vi "Logging Message Loop.vi"(8 "error in (no error)":errorcluster, 10 "data queue in":refnum<queue>, 11 "Message Queues":T1) -> (0 "error out":errorcluster)   [LabVIEW 2026, in "Logging.lvlib"]
doc: "The message loop subVI to handle messages pertaining to logging data."
uses:
  Logging.lvlib
  support/Message Queue/All Message Queues.ctl
  support/Message Queue/Message Cluster.ctl
  controls/NotifierAndDataQueue.ctl
  controls/WaveformChartData.ctl
  Logging Configuration.ctl
  Logging State.ctl
  support/Message Queue/Enqueue Message (Single).vi
  <vilib>/Utility/error.llb/Error Cluster From Error Code.vi
  <vilib>/ErrorRing/Error Ring.xnode
  support/Message Queue/Message Queue.lvlib
  Settings/Settings.lvlib
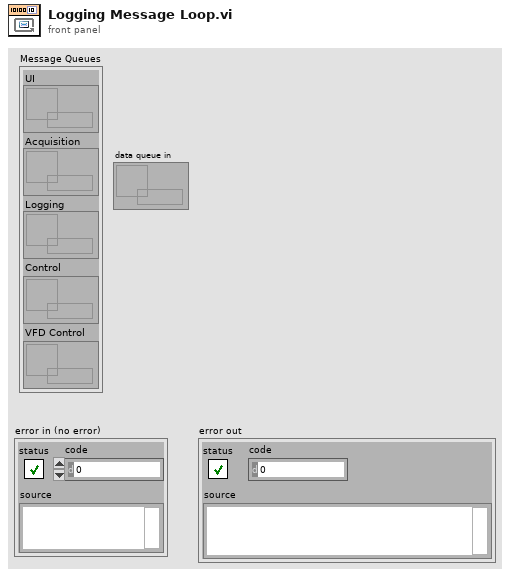
[diagram p1: front panel]
types:
  T1 = typedef "Message Queue.lvlib/All Message Queues.ctl" = cluster{"UI":refnum<queue>, "Acquisition":refnum<queue>, "Logging":refnum<queue>, "Control":refnum<queue>, "VFD Control":refnum<queue>}
  T2 = typedef "Logging.lvlib/Logging State.ctl" = cluster{"State":enum16{"Logging", "Not Logging", "Idle"}, "Samples to Save":u32, "Force Trigger":bool}
  T3 = typedef "Logging.lvlib/Logging Configuration.ctl" = cluster{"Log File Base Path":path, "TDMS File Reference":refnum<k34>, "File Name":string, "Headers To Write":string[]}
  T4 = enum16{"open", "open or create", "create or replace", "create", "open (read-only)"}
  T5 = typedef "NotifierAndDataQueue.ctl" = cluster{"Ai0":dbl, "Ai1":dbl, "Ai2":dbl, "Ai3":dbl, "Ai4":dbl, "Ai5":dbl, "Ai6":dbl, "Ai7":dbl, "Belt Slip?":bool, "P0.1":bool, "P0.2":bool, "P0.3":bool, "P0.4":bool, "P0.5":bool, "P0.6":bool, "P0.7":bool, "2D Numeric Data":dbl[][], "String 2":string, "String 1":string, "Waveform Chart Data":T6, "Live Pulley Ratio":dbl, "Data Table":string[][]}
  T6 = typedef "Settings.lvlib/WaveformChartData.ctl" = cluster{"DUT Vacuum":dbl, "Motor RPM":dbl, "DUT RPM":dbl, "Tank Vacuum":dbl}
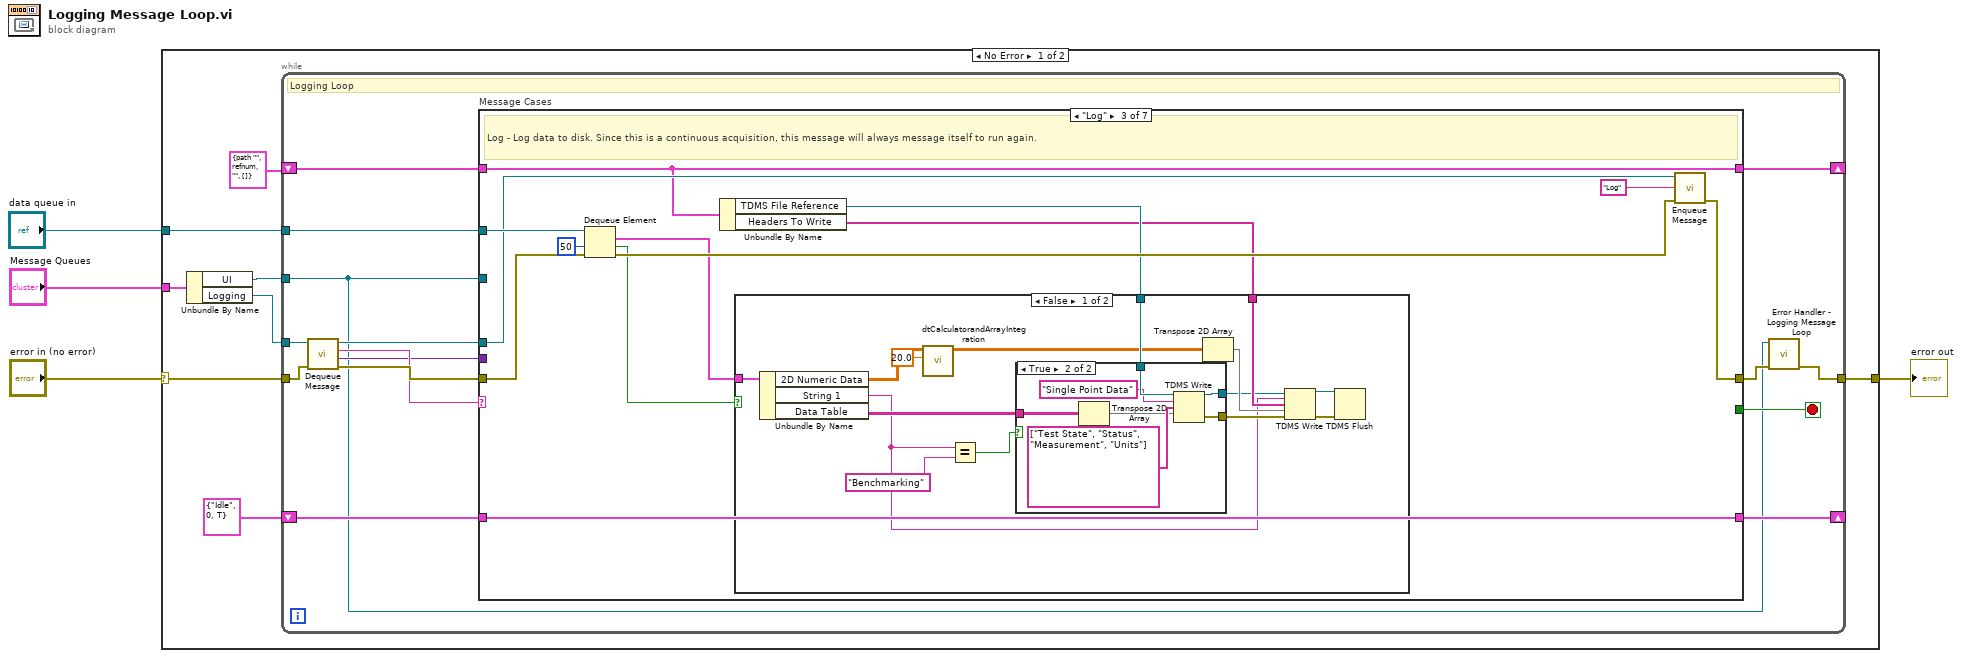
[diagram p0: block diagram]
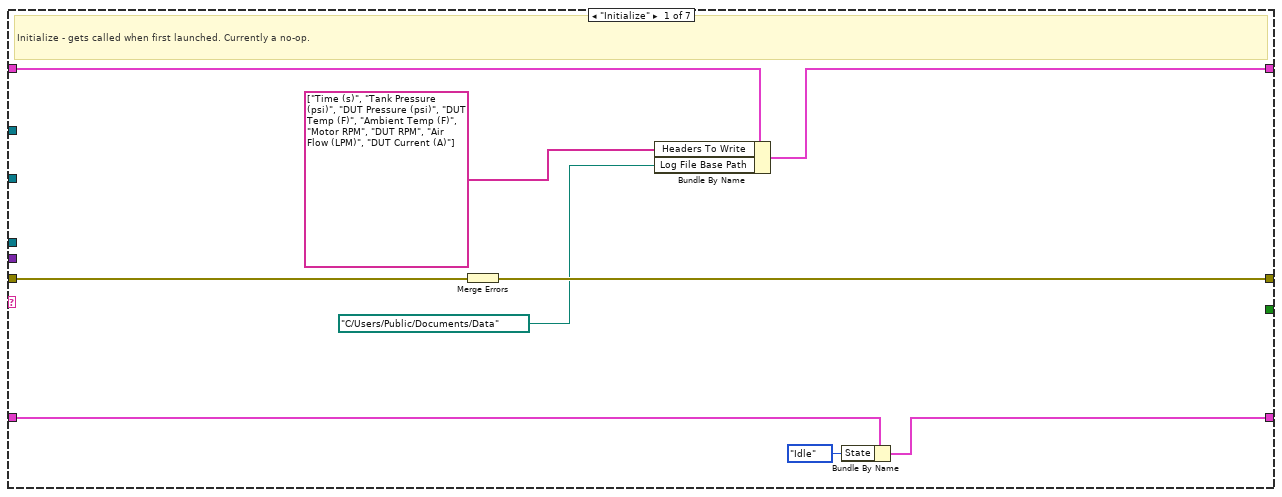
[diagram p2: hidden frame]
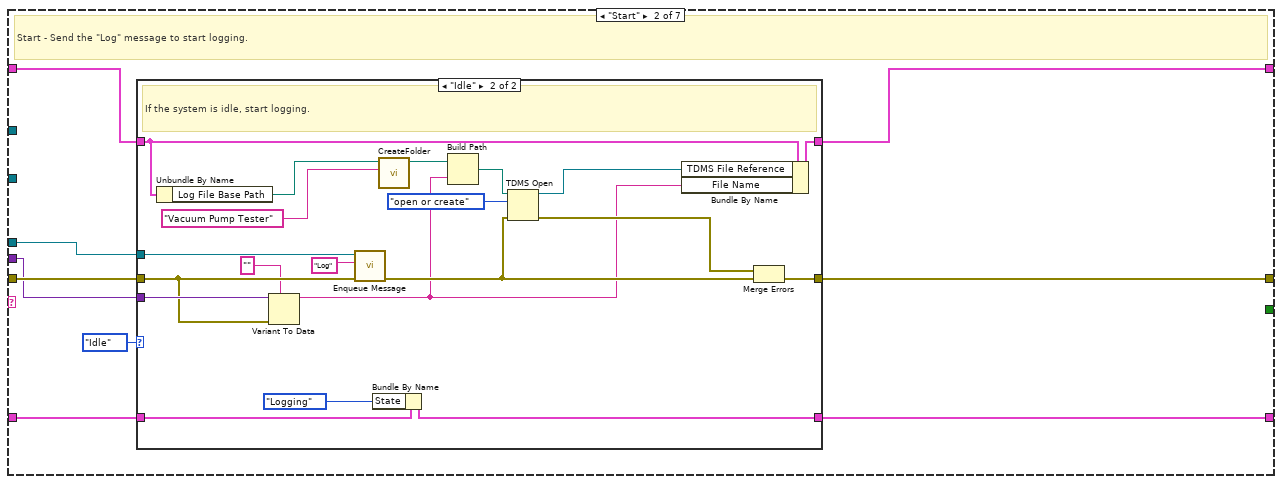
[diagram p3: hidden frame]
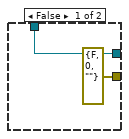
[diagram p5: hidden frame]
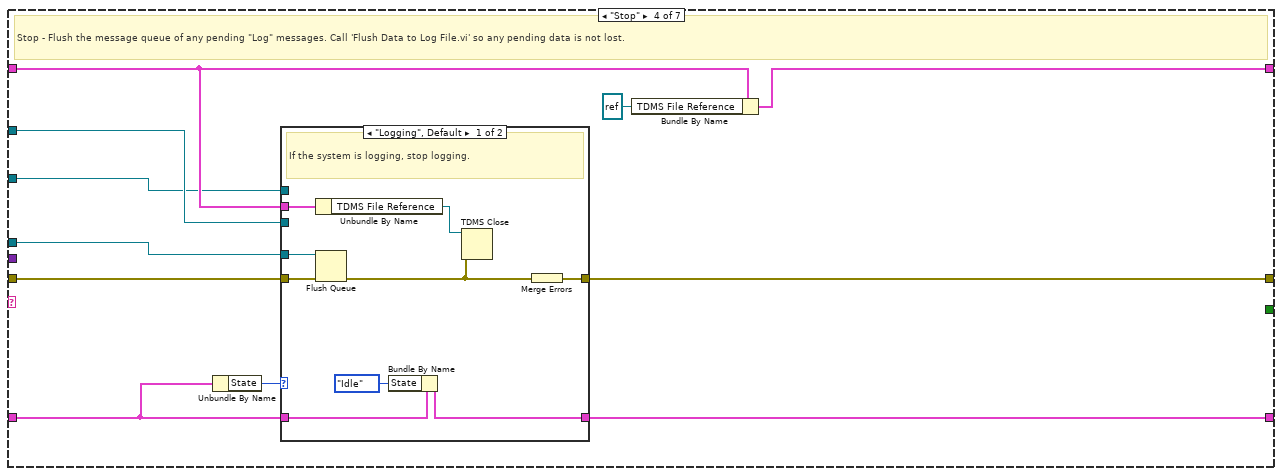
[diagram p7: hidden frame]
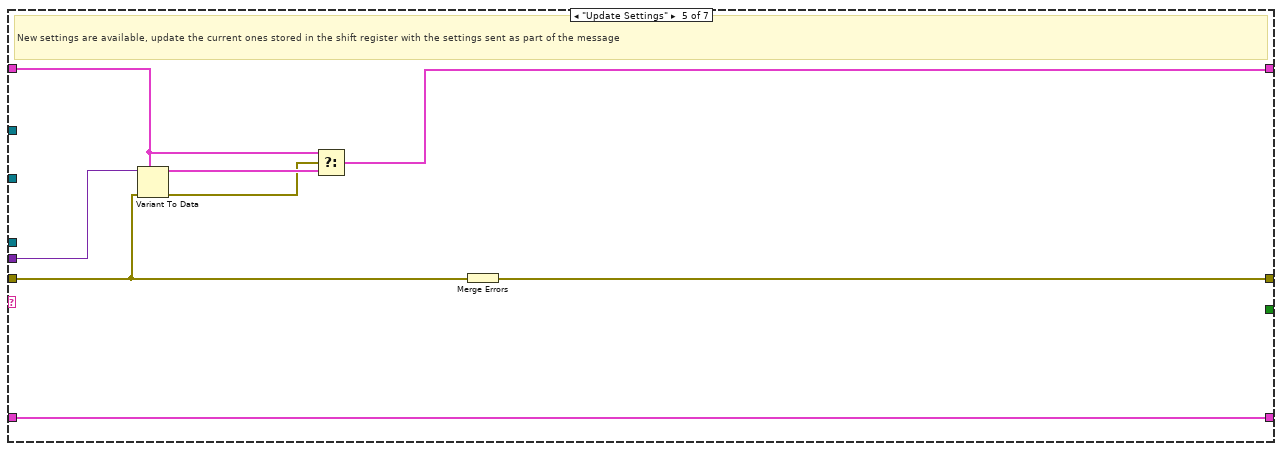
[diagram p9: hidden frame]
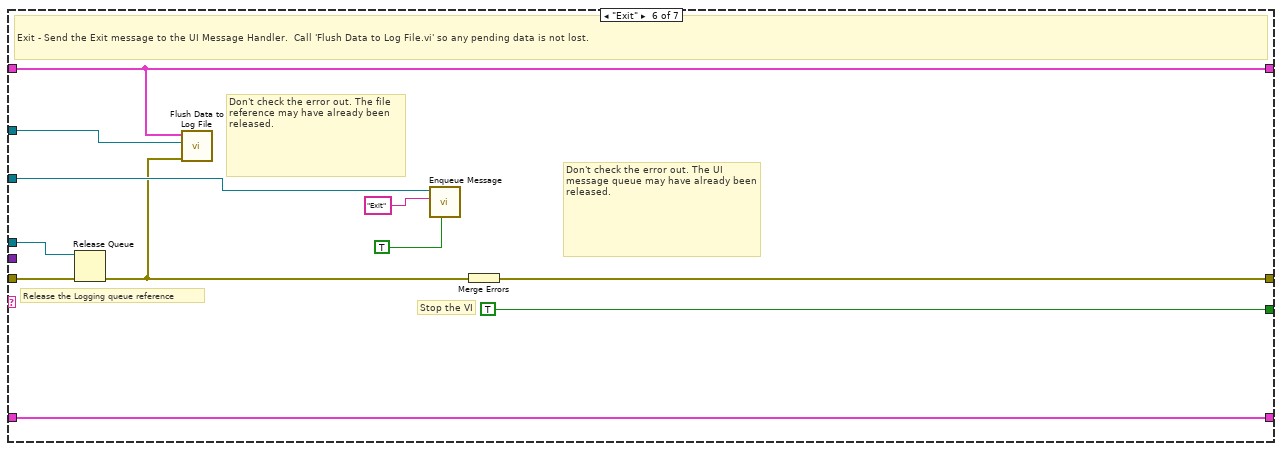
[diagram p10: hidden frame]
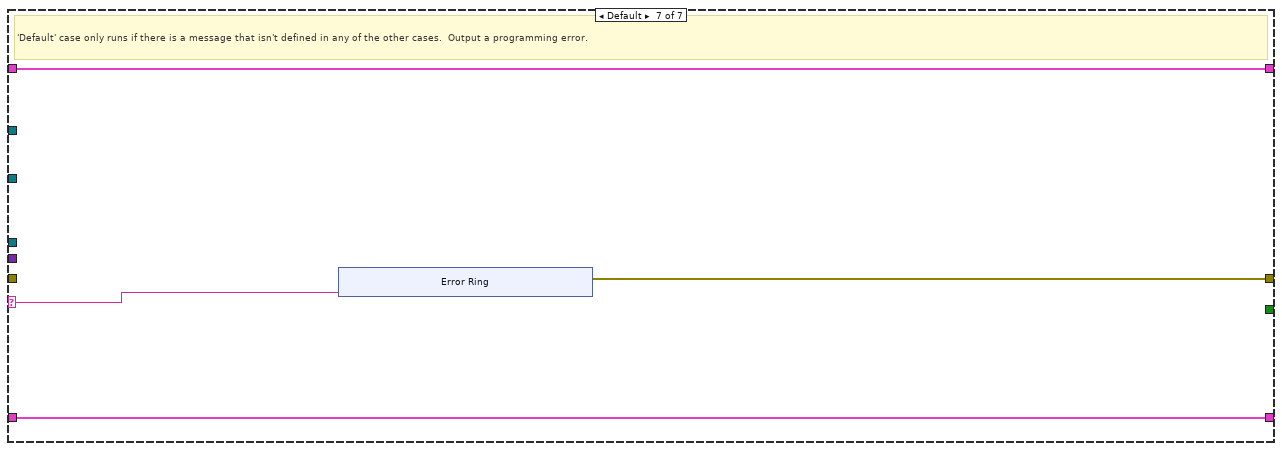
[diagram p11: hidden frame]
diagram:
  n1 = case shown="No Error" "error in (no error)" {
    selector: "error in (no error)" -> [w8 w158]
    tunnel: "Message Queues" -> [w12 _]
    tunnel: [w10 w158] -> w3
    tunnel: "data queue in" -> [w7 _]
    frame No Error {
      n2 = Unbundle By Name(w12) -> ("UI"=w6:refnum<queue>, "Logging"=w11:refnum<queue>)
      n3 = while {
        tunnel: w11 -> [w19]
        shift-right: [w26] -> _
        shift-left: T3 {"Log File Base Path"=path "", "TDMS File Reference"=refnum, "File Name"="", "Headers To Write"=[]} ("Logging Configuration") -> [w27]
        tunnel: w6 -> [w14]
        tunnel: w7 -> [w13]
        shift-right: [w17] -> _
        shift-left: T2 {"State"=enum."Idle", "Samples to Save"=0, "Force Trigger"=TRUE} -> [w18]
        tunnel: w8 -> [w24]
        tunnel: [w15] -> w10
        stop <- w25 stop-if-true
        # "Logging Loop"
        n4 = call "Dequeue Message.vi"("error in (no error)"=w24, "Message Queue"=w19) -> ("error out"=w23:errorcluster, "Message Data"=w21:variant, "Message"=w22:string, "dup Message Queue"=w20:refnum<queue>)  [unwired: 6 in]
        n5 = case "Message Cases" shown="\"Log\"" w22 {
          selector: w22 -> [_ _ _ _ _ _ w147]
          tunnel: w20 -> [_ w44 w77 w114 _ w140 _]
          tunnel: w23 -> [w35 w43 w79 w115 w129 w143 _]
          tunnel: [w36 w45 w81 w116 w135 w145 w148] -> w16
          tunnel: w27 -> [w31 w42 w74 w111 w133 w139 w150]
          tunnel: [w30 w41 w74 w113 w130 w139 w150] -> w26
          tunnel: [_ _ _ _ _ TRUE _] -> w25
          tunnel: w21 -> [_ w38 _ _ w134 _ _]
          tunnel: w14 -> [_ _ _ w109 _ w144 _]
          tunnel: w13 -> [_ _ w78 w110 _ w136 _]
          tunnel: w18 -> [w34 w39 w76 w107 w128 w137 w149]
          tunnel: [w33 w40 w76 w106 w128 w137 w149] -> w17
          frame "Initialize" {
            # "Initialize - gets called when first launched. Currently a no-op."
            n6 = Merge Errors(w35) -> (w36:errorcluster)
            n7 = Bundle By Name(cluster=w31, "Headers To Write"=string[] ["Time (s)", "Tank Pressure (psi)", "DUT Pressure (psi)", "DUT Temp (F)", "Ambient Temp (F)", "Motor RPM", "DUT RPM", "Air Flow (LPM)", "DUT Current (A)"], "Log File Base Path"=path "C:/Users/Public/Documents/Data") -> (w30:T3)
            n8 = Bundle By Name(cluster=w34, "State"=enum16{"Logging", "Not Logging", "Idle"}."Idle") -> (w33:T2)
          }
          frame "Start" {
            # "Start - Send the \"Log\" message to start logging."
            n9 = case shown="\"Idle\"" enum16{"Logging", "Not Logging", "Idle"}."Idle" ("State") {
              tunnel: [w47 w68] -> w45
              tunnel: w44 -> [_ w67]
              tunnel: w43 -> [w47 w52]
              tunnel: w42 -> [w48 w65]
              tunnel: [w48 w62] -> w41
              tunnel: w39 -> [w46 w58]
              tunnel: [w46 w57] -> w40
              tunnel: w38 -> [_ w53]
              frame "Logging", Default {
                # "The system is already running. Ignore the \"Start\" message."
              }
              frame "Idle" {
                # "If the system is idle, start logging."
                n10 = Unbundle By Name(w65) -> ("Log File Base Path"=w55:path)
                n11 = Variant To Data(error in=w52, type="", Variant=w53) -> (data=w50:string)  [unwired: 1 out]
                n12 = call-poly "Enqueue Message.vi"("error in (no error)"=w52, "Message"="Log", "Message Queue"=w67) -> ("error out"=w60:errorcluster)  [unwired: 7 in, 1 out]
                n13 = Bundle By Name(cluster=w58, "State"=enum16{"Logging", "Not Logging"}."Logging") -> (w57:T2)
                n14 = call "CreateFolder.vi"("Folder Name"="Vacuum Pump Tester", "path (use dialog)"=w55) -> ("created path"=w54:path)  [unwired: 9 in]
                n15 = Build Path(base path=w54, name or relative path=w50) -> (appended path=w63:path)
                n16 = TDMS Open(8:w60, 10:T4."open or create" ("operation (0:open)"), 11:w63) -> (0:w59:errorcluster, 3:w64:refnum<k34>)  [unwired: 4 in]
                n17 = Bundle By Name(cluster=w65, "TDMS File Reference"=w64, "File Name"=w50) -> (w62:T3)
                n18 = Merge Errors(w59, w60) -> (w68:errorcluster)
              }
            }
          }
          frame "Log" {
            # "Log - Log data to disk. Since this is a continuous acquisition, this message will always message itself to run again."
            n19 = Dequeue Element(queue=w78, timeout in ms (-1)=50, error in (no error)=w79) -> (element=w73:T5, timed out?=w70:bool, error out=w75:errorcluster)  [unwired: 1 out]
            n20 = Unbundle By Name(w74) -> ("TDMS File Reference"=w72:refnum<k34>, "Headers To Write"=w69:string[])
            n21 = case shown="False" w70 {
              tunnel: w73 -> [w95 _]
              tunnel: w72 -> [w91 _]
              tunnel: w69 -> [w96 _]
              frame False {
                n22 = Unbundle By Name(w95) -> ("2D Numeric Data"=w87:dbl[][], "String 1"=w83:string, "Data Table"=w88:string[][])
                n23 = call "dtCalculatorandArrayIntegration.vi"("Sampling Rate"=20.0, "Data Input"=w87) -> ("output array"=w86:dbl[][])  [unwired: 9 in]
                n24 = Equal?(x=w83, y="Benchmarking") -> (x = y?=w84:bool)
                n25 = case shown="True" w84 {
                  tunnel: w91 -> [w98 w105]
                  tunnel: [w98 w104] -> w90
                  tunnel: [errorcluster {"status"=FALSE, "code"=0, "source"=""} ("error out") w103] -> w89
                  tunnel: w88 -> [_ w101]
                  frame False {
                  }
                  frame True {
                    n26 = Transpose 2D Array(2D array=w101) -> (transposed array=w99:string[][])
                    n27 = TDMS Write(0:w105, 5:"Single Point Data" ("group name in (Untitled)"), 7:string[] ["Test State", "Status", "Measurement", "Units"] ("Headers To Write"), 9:w99) -> (4:w104:refnum<k34>, 15:w103:errorcluster)  [unwired: 2 in, 2 out]
                  }
                }
                n28 = Transpose 2D Array(2D array=w86) -> (transposed array=w92:dbl[][])
                n29 = TDMS Write(0:w90, 5:w83, 7:w96, 9:w92, 11:w89) -> (4:w93:refnum<k34>, 15:w94:errorcluster)  [unwired: 1 in, 2 out]
                n30 = TDMS Flush(4:w94, 7:w93) -> ()  [unwired: 2 out]
              }
              frame True {
              }
            }
            n31 = call-poly "Enqueue Message.vi"("error in (no error)"=w75, "Message"="Log", "Message Queue"=w77) -> ("error out"=w81:errorcluster)  [unwired: 7 in, 1 out]
          }
          frame "Stop" {
            # "Stop - Flush the message queue of any pending \"Log\" messages. Call 'Flush Data to Log File.vi' so any pending data is not lost."
            n32 = Unbundle By Name(w107) -> ("State"=w108:enum16{"Logging", "Not Logging", "Idle"})
            n33 = case shown="\"Logging\", Default" w108 {
              tunnel: [w125 w127] -> w116
              tunnel: w115 -> [w124 w127]
              tunnel: w114 -> [w123 _]
              tunnel: w111 -> [w118 _]
              tunnel: w110 -> [_ _]
              tunnel: w109 -> [_ _]
              tunnel: w107 -> [w122 w126]
              tunnel: [w121 w126] -> w106
              frame "Logging", Default {
                # "If the system is logging, stop logging."
                n34 = Unbundle By Name(w118) -> ("TDMS File Reference"=w117:refnum<k34>)
                n35 = Flush Queue(queue=w123, error in (no error)=w124) -> (error out=w119:errorcluster)  [unwired: 2 out]
                n36 = Bundle By Name(cluster=w122, "State"=enum16{"Logging", "Not Logging", "Idle"}."Idle") -> (w121:T2)
                n37 = TDMS Close(8:w119, 11:w117) -> ()  [unwired: 2 out]
                n38 = Merge Errors(w119) -> (w125:errorcluster)
              }
              frame "Idle" {
                # "The system is already idle. Ignore the \"Stop\" message."
              }
            }
            n39 = Bundle By Name(cluster=w111, "TDMS File Reference"=refnum<k34> refnum ("tdms file out")) -> (w113:T3)
          }
          frame "Update Settings" {
            # "New settings are available, update the current ones stored in the shift register with the settings sent as part of the message"
            n40 = Variant To Data(error in=w129, type=w133, Variant=w134) -> (data=w132:T3, error out=w131:errorcluster)
            n41 = Select(t=w133, s=w131, f=w132) -> (s? t:f=w130:T3)
            n42 = Merge Errors(w129) -> (w135:errorcluster)
          }
          frame "Exit" {
            # "Don't check the error out. The file reference may have already been released."
            # "Release the Logging queue reference"
            # "Don't check the error out. The UI message queue may have already been released."
            # "Stop the VI"
            # "Exit - Send the Exit message to the UI Message Handler.  Call 'Flush Data to Log File.vi' so any pending data is not lost."
            n43 = Release Queue(queue=w140, error in (no error)=w143) -> (error out=w138:errorcluster)  [unwired: 1 in, 2 out]
            n44 = call "Flush Data to Log File.vi"("error in (no error)"=w138, "data queue in"=w136, "Logging Configuration"=w139) -> ()  [unwired: 8 in, 1 out]
            n45 = call-poly "Enqueue Message.vi"("Priority Message? (F)"=TRUE, "Message"="Exit", "Message Queue"=w144) -> ()  [unwired: 7 in, 2 out]
            n46 = Merge Errors(w138) -> (w145:errorcluster)
          }
          frame Default {
            # "'Default' case only runs if there is a message that isn't defined in any of the other cases.  Output a programming error."
            n47 = xnode "Error Ring"("parameter 0"=w147) -> ("error out"=w148:errorcluster)
          }
        }
        n48 = call "Error Handler - Logging Message Loop.vi"("error in (no error)"=w16, "Message Queue"=w14) -> ("dup error in"=w15:errorcluster)  [unwired: 8 in, 1 out]
      }
    }
    frame Error {
    }
  }
  "error out" <- w3
